vi "unbundle config parse cmd.vi"(11 "Parsed CMD":T1) -> (1 "Value string":string, 2 "Command":string, 3 "Channel number not index":i32, 4 "Value double":dbl)   [LabVIEW 2020]
uses:
  parsed device cmd.ctl
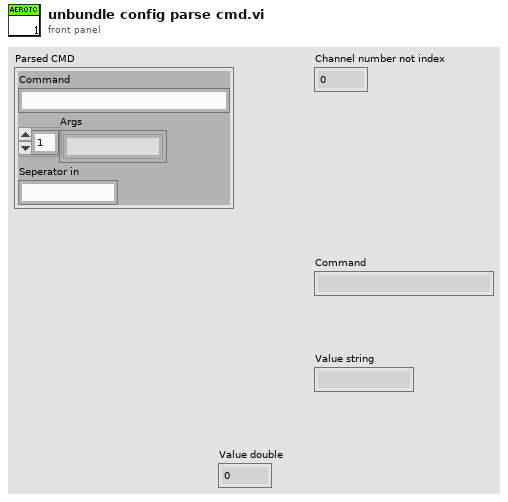
[diagram p1: front panel]
types:
  T1 = typedef "parsed device cmd.ctl" = cluster{"Command":string, "Args":string[], "Seperator in":string}
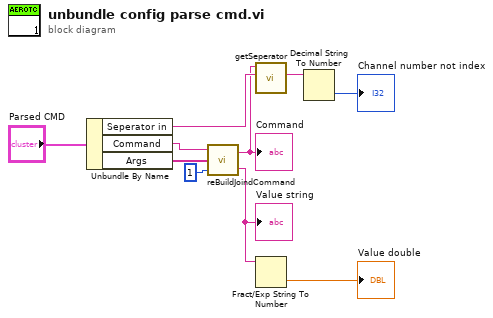
[diagram p0: block diagram]
diagram:
  n1 = Unbundle By Name("Parsed CMD") -> ("Seperator in"=w9:string, "Command"=w8:string, "Args"=w10:string[])
  n2 = call "reBuildJoindCommand.vi"("number of group elements (0)"=1, "Args"=w10, "Command 2"=w8) -> ("Arg"=w4:string, "Command"=w5:string)
  "Command" <- w5
  "Value string" <- w4
  n3 = call "getSeperator.vi"("Channel Seperator (\"\")"=w9, "Command"=w5) -> ("Channel"=w2:string)  [unwired: 8 in, 1 out]
  n4 = Fract/Exp String To Number(string=w4) -> (number=→"Value double":dbl)  [unwired: 3 in, 1 out]
  n5 = Decimal String To Number(string=w2) -> (number=→"Channel number not index":i32)  [unwired: 2 in, 1 out]
